vi "Cache Config Info.vi"(8 "error in (no error)":errorcluster, 11 "System Config Server in":refnum<class "System Config Module.lvclass">) -> (0 "error out":errorcluster, 3 "System Config Server out":refnum<class "System Config Module.lvclass">)   [LabVIEW 2020, in "Volatus.lvlib" / "System Config Module.lvclass"]
uses:
  System Config Module.lvclass
  C:/dev/lv20CE/relink/lv-volatus/Volatus/Module/Module.lvclass
  Module/Module.lvclass/Module.ctl
  VolatusAPI/VolatusAPI.lvclass/VolatusAPI.ctl
  System Config Module.lvclass/System Config Module.ctl
  Module/Module.lvclass
  VolatusAPI/VolatusAPI.lvclass
  VolatusConfig/Node/Node Config.lvclass
  lv-vecto/Vecto/Node Config/Node Config.lvclass
  lv-builder/Builder Core/Builder Core.lvlib
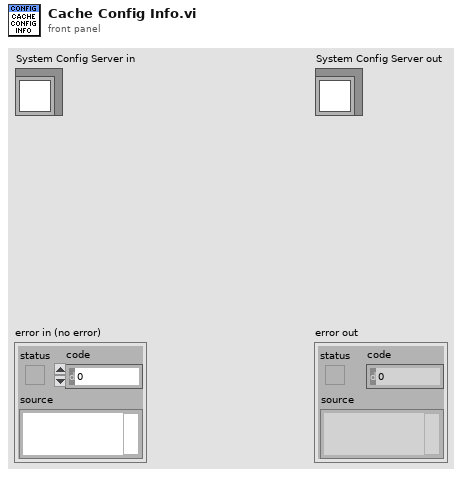
[diagram p1: front panel]
types:
  T1 = typedef "Builder Core.lvlib/Version.ctl" = cluster{"Major":u16, "Minor":u16, "Fix":u16, "Build":u16}
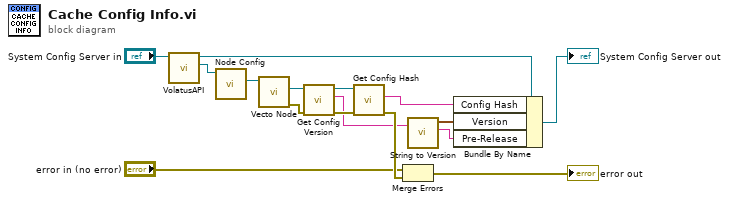
[diagram p0: block diagram]
diagram:
  n1 = call "VolatusAPI.vi"("Module in"="System Config Server in") -> ("VolatusAPI"=w11:refnum<class "VolatusAPI.lvclass">, "Module out"=w2:refnum<class "System Config Module.lvclass">)  [unwired: 9 in]
  n2 = call "Node Config.vi"("VolatusAPI in"=w11) -> ("Node Config"=w10:refnum<class "Node Config.lvclass">)  [unwired: 9 in, 1 out]
  n3 = call "Vecto Node.vi"("Node in"=w10) -> ("error out"=w8:errorcluster, "Vecto Node"=w9:refnum<class "Node Config.lvclass">)  [unwired: 8 in, 1 out]
  n4 = call "Get Config Version.vi"("error in (no error)"=w8, "Node Config in"=w9) -> ("error out"=w15:errorcluster, "Config Version"=w5:string, "Node Config out"=w4:refnum<class "Node Config.lvclass">)  [unwired: 7 in]
  n5 = call "Get Config Hash.vi"("error in (no error)"=w15, "Node Config in"=w4) -> ("error out"=w16:errorcluster, "Config Hash"=w3:string)  [unwired: 7 in, 1 out]
  n6 = Merge Errors("error in (no error)", w16) -> (→"error out":errorcluster)
  n7 = call "String to Version.vi"("Version String"=w5) -> ("Version"=w7:T1, "Pre-Release"=w6:string)  [unwired: 4 in, 1 out]
  n8 = Bundle By Name(cluster=w2, "Config Hash"=w3, "Version"=w7, "Pre-Release"=w6) -> (→"System Config Server out":refnum<class "System Config Module.lvclass">)
